vi "Configure Device.vi"(8 "error in (no error)":errorcluster, 10 "Max beams":dbl, 11 "Maxscend SP4T in":refnum<class "Maxscend SP4T.lvclass">) -> (0 "error out":errorcluster, 3 "Maxscend SP4T out":refnum<class "Maxscend SP4T.lvclass">)   [LabVIEW 2020, in "Maxscend SP4T.lvclass"]
uses:
  Maxscend SP4T.lvclass
panel:
  in  "All":bool
  in  "Truth Table":T1(array[cluster])=[{"Enabled"=TRUE, "State"=1.0, "V1 V2 V3"=[FALSE, FALSE, TRUE], "RF Path"="All Ron"}, {"Enabled"=TRUE, "State"=2.0, "V1 V2 V3"=[FALSE, TRUE, TRUE], "RF Path"="ANT to RF1 and RF2"}, {"Enabled"=TRUE, "State"=3.0, "V1 V2 V3"=[TRUE, FALSE, TRUE], "RF Path"="ANT to RF3 and RF4"}, {"Enabled"=TRUE, "State"=4.0, "V1 V2 V3"=[FALSE, FALSE, FALSE], "RF Path"="ANT to RF1"}, {"Enabled"=TRUE, "State"=5.0, "V1 V2 V3"=[FALSE, TRUE, FALSE], "RF Path"="ANT to RF2"}, {"Enabled"=TRUE, "State"=6.0, "V1 V2 V3"=[TRUE, FALSE, FALSE], "RF Path"="ANT to RF3"}, {"Enabled"=TRUE, "State"=7.0, "V1 V2 V3"=[TRUE, TRUE, FALSE], "RF Path"="ANT to RF4"}, {"Enabled"=TRUE, "State"=8.0, "V1 V2 V3"=[TRUE, TRUE, TRUE], "RF Path"="All isolation"}]
  in  "DAQmx line names":T2(array[cluster])=[{"lines"="Dev2/port0/line0", "Function"="Ctrl1", "Function"=enum."Control 1"}, {"lines"="Dev2/port1/line5", "Function"="Ctrl2", "Function"=enum."Control 2"}, {"lines"="Dev2/port2/line4", "Function"="Ctrl3", "Function"=enum."Control 3"}]
  in  "Cancel Button":bool
  in  "OK Button":bool
  # "V1    V2     V3"
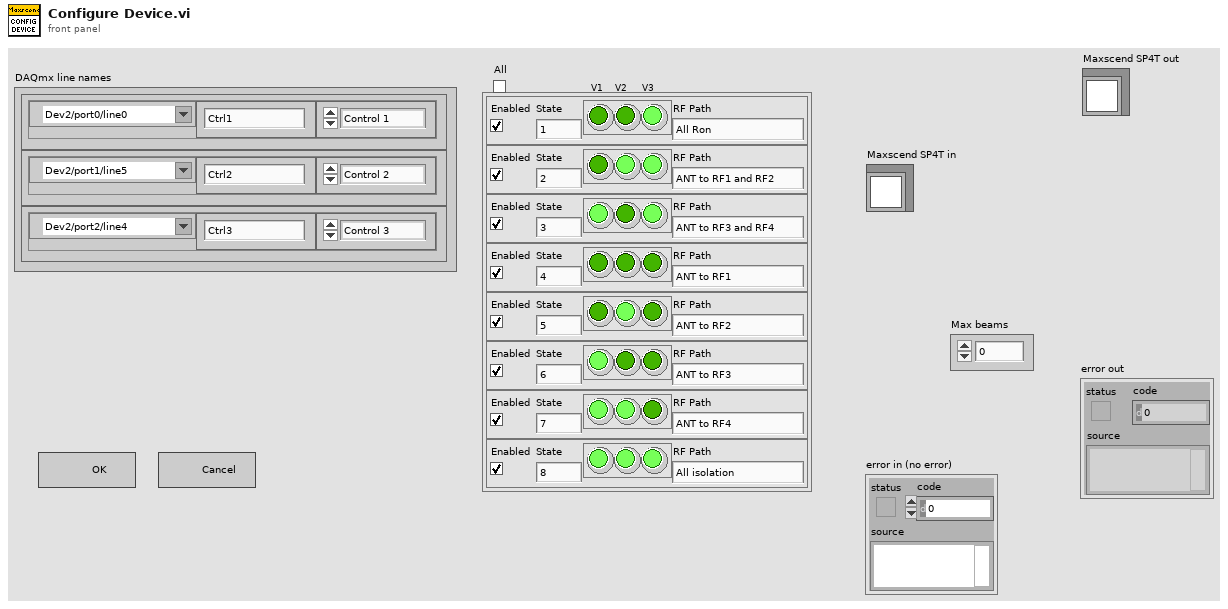
[diagram p1: front panel]
types:
  T1 = cluster{"Enabled":bool, "State":dbl, "V1 V2 V3":bool[], "RF Path":string}[]
  T2 = cluster{"lines":tag, "Function":string, "Function":enum16{"Vdd", "Control 0", "Control 1", "Control 2", "Control 3"}}[]
  T3 = cluster{"Enabled":bool, "State":dbl, "V1 V2 V3":bool[], "RF Path":string}
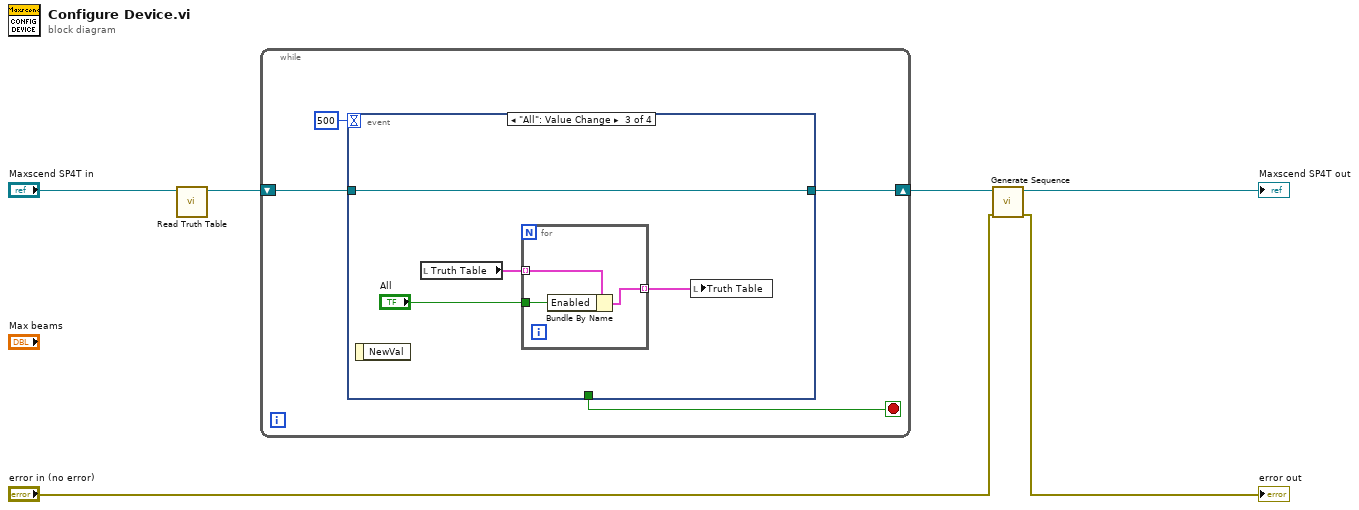
[diagram p0: block diagram]
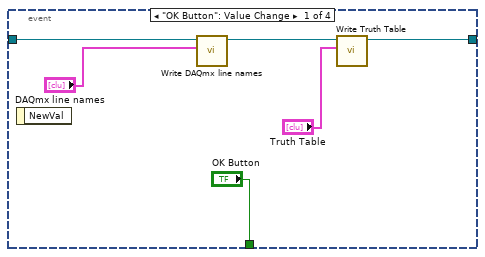
[diagram p2: hidden frame]
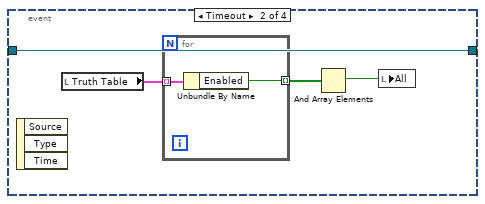
[diagram p3: hidden frame]
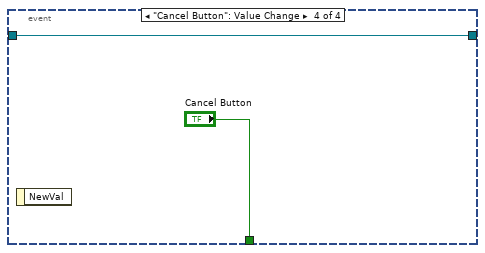
[diagram p4: hidden frame]
diagram:
  n1 = call-dynamic "Read Truth Table.vi"("Maxscend SP4T in"="Maxscend SP4T in") -> ("Maxscend SP4T out"=w5:refnum<class "Maxscend SP4T.lvclass">)  [unwired: 9 in, 1 out]
  n2 = while {
    shift-right: [w8] -> w4
    shift-left: w5 -> [w9]
    stop <- w10 stop-if-true
    n3 = event shown="[2] \"All\": Value Change" {
      selector: _ -> [_ _ _ _]
      dyn-events: _ -> [_ _ _ _]
      timeout: 500 -> [_ _ _ _]
      tunnel: ["OK Button" _ _ "Cancel Button"] -> w10
      tunnel: w9 -> [w13 w20 w26 w30]
      tunnel: [w14 w20 w26 w30] -> w8
      event "OK Button": Value Change {
        n4 = event-data() -> ()  [unwired: 1 in, 1 out]
        n5 = call-dynamic "Write DAQmx line names.vi"("DAQmx line names"="DAQmx line names", "NI DAQmx in"=w13) -> ("NI DAQmx out"=w12:refnum<class "Maxscend SP4T.lvclass">)  [unwired: 8 in, 1 out]
        n6 = call-dynamic "Write Truth Table.vi"("Truth Table"="Truth Table", "Maxscend SP4T in"=w12) -> ("Maxscend SP4T out"=w14:refnum<class "Maxscend SP4T.lvclass">)  [unwired: 9 in]
      }
      event Timeout {
        n7 = event-data() -> ()  [unwired: 1 in, 3 out]
        n8 = local read "Truth Table"() -> (w19:T1)
        n9 = for {
          tunnel: w19 -> [w22] mode=indexing
          tunnel: [w21] -> w18 mode=indexing
          n10 = Unbundle By Name(w22) -> ("Enabled"=w21:bool)
        }
        n11 = And Array Elements(Boolean array=w18) -> (logical AND=w17:bool)
        n12 = local write "All"(w17) -> ()
      }
      event "All": Value Change {
        n13 = event-data() -> ()  [unwired: 1 in, 1 out]
        n14 = local read "Truth Table"() -> (w25:T1)
        n15 = for {
          tunnel: w25 -> [w29] mode=indexing
          tunnel: "All" -> [w28]
          tunnel: [w27] -> w23 mode=indexing
          n16 = Bundle By Name(cluster=w29, "Enabled"=w28) -> (w27:T3)
        }
        n17 = local write "Truth Table"(w23) -> ()
      }
      event "Cancel Button": Value Change {
        n18 = event-data() -> ()  [unwired: 1 in, 1 out]
      }
    }
  }
  n19 = call-dynamic "Generate Sequence.vi"("error in (no error)"="error in (no error)", "Maxscend SP4T in"=w4) -> ("error out"=→"error out":errorcluster, "Maxscend SP4T out"=→"Maxscend SP4T out":refnum<class "Maxscend SP4T.lvclass">)  [unwired: 8 in]
